vi "Get Whole Image.vi"(9 "Frame Num":u16, 10 "Images":T2, 11 "2D Picture in":picture) -> (3 "2D Picture out":picture)   [LabVIEW 2021, in "NI Measurement Plug-In SDK.lvlib" / "VI Info.lvlib"]
doc: "This VI uses the Owner Index field to draw all the background block diagram information for a given frame, for use in the Preview Window."
uses:
  VI Info.lvlib
  <vilib>/picture/picture.llb/imagedata.ctl
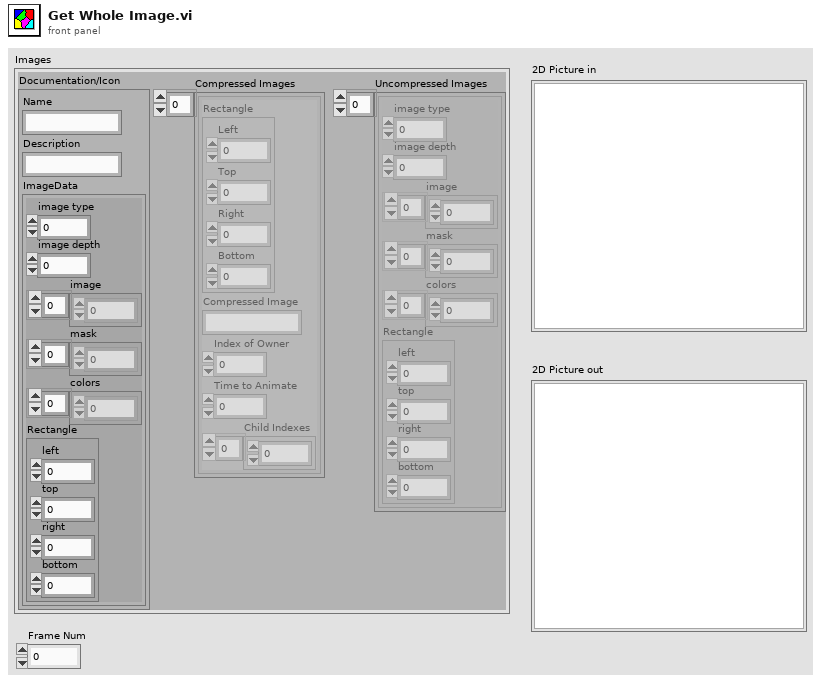
[diagram p1: front panel]
types:
  T1 = typedef "imagedata.ctl" = cluster{"image type":i32, "image depth":i32, "image":u8[], "mask":u8[], "colors":u32[], "Rectangle":cluster{"left":i16, "top":i16, "right":i16, "bottom":i16}}
  T2 = cluster{"Documentation/Icon":cluster{"Name":string, "Description":string, "ImageData":T1}, "Compressed Images":cluster{"Rectangle":cluster{"Left":i32, "Top":i32, "Right":u32, "Bottom":u32}, "Compressed Image":string, "Index of Owner":i32, "Time to Animate":i32, "Child Indexes":i32[]}[], "Uncompressed Images":T1[]}
  T3 = cluster{"Rectangle":cluster{"Left":i32, "Top":i32, "Right":u32, "Bottom":u32}, "Compressed Image":string, "Index of Owner":i32, "Time to Animate":i32, "Child Indexes":i32[]}[]
  T4 = cluster{"Rectangle":cluster{"Left":i32, "Top":i32, "Right":u32, "Bottom":u32}, "Compressed Image":string, "Index of Owner":i32, "Time to Animate":i32, "Child Indexes":i32[]}
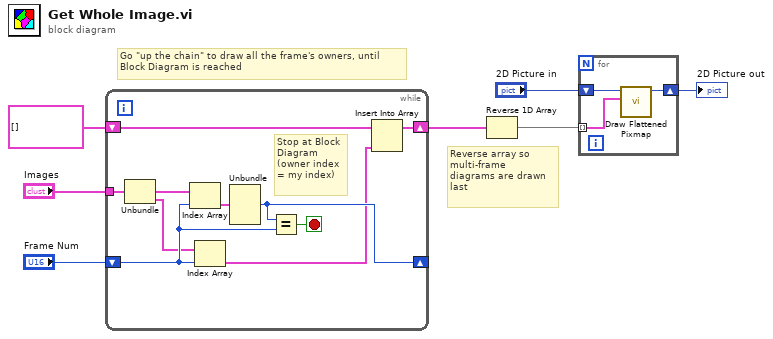
[diagram p0: block diagram]
diagram:
  # "Reverse array so \nmulti-frame \ndiagrams are drawn \nlast"
  # "Go \"up the chain\" to draw all the frame's owners, until\nBlock Diagram is reached"
  n1 = while {
    tunnel: "Images" -> [w16]
    shift-right: [w14] -> _
    shift-left: "Frame Num" -> [w13]
    shift-right: [w11] -> w1
    shift-left: T1[] [] -> [w12]
    stop <- w15 stop-if-true
    # "Stop at Block\nDiagram\n(owner index\n= my index)"
    n2 = Unbundle(w16) -> ("Compressed Images"=w10:T3, "Uncompressed Images"=w9:T1[])  [unwired: 1 out]
    n3 = Index Array(array=w10, index=w13) -> (element=w17:T4)
    n4 = Index Array(array=w9, index=w13) -> (element=w8:T1)
    n5 = Unbundle(w17) -> ("Index of Owner"=w14:i32)  [unwired: 4 out]
    n6 = Equal?(x=w14, y=w13) -> (x = y?=w15:bool)
    n7 = Insert Into Array(array=w12, new element=w8) -> (w11:T1[])  [unwired: 1 in]
  }
  n8 = Reverse 1D Array(array=w1) -> (reversed array=w2:T1[])
  n9 = for {
    tunnel: w2 -> [w19] mode=indexing
    shift-right: [w18] -> w5
    shift-left: "2D Picture in" -> [w20]
    n10 = call <vilib>:"Draw Flattened Pixmap.vi"("image data"=w19, "picture"=w20) -> ("new picture"=w18:picture)  [unwired: 7 in]
  }
  "2D Picture out" <- w5
